vi "KeyDown.vi"(6 "PlatMods":T9, 7 "Type":T1, 8 "error in (no error)":errorcluster, 9 "VKey":T10, 10 "Char":i16, 11 "Data in":T2={"Class"={"Ants"=refnum, "Layer"=refnum, "Templates"=refnum, "Icon"=refnum, "Glyph"=refnum, "Settings"=refnum, "Tools"=refnum, "History"=refnum}, "Ref"={"Add Layer"=refnum, "Remove Layer"=refnum, "Line Text"=[], "Body Text Spec"=refnum, "DNL_Font"=refnum, "glyph path str"=refnum, "templates path str"=refnum, "Arrow Up"=refnum, "Arrow Down"=refnum, "IE VI Ref"=refnum, "Glyphs tree"=refnum, "Templates tree"=refnum, "Layer Icon Text"=refnum, "Layer Template"=refnum, "Body Text"=refnum, "Search Templates"=refnum, "TextMarker"=refnum, "Tab Control"=refnum, "Search Glyphs"=refnum, "Line Color"=refnum, "DNL_Glyphs []"=refnum, "Fill Color"=refnum, "Tools"=refnum, "Icon"=refnum, "Preview"=refnum, "Ants"=refnum, "Terminals"=refnum, "menu reference"=refnum, "LayerNames"=[], "GlyphLoadAnimation"=refnum, "TemplateLoadAnimation"=refnum, "refreshGlyphs"=refnum, "refreshTemplates"=refnum}, "Support"={"AntsRect"={"left"=0, "top"=0, "right"=0, "bottom"=0}, "Mouse Move Coords"={"Horizontal"=0, "Vertical"=0}, "Mouse Down Coords"={"Horizontal"=0, "Vertical"=0}, "Temp Coord"={"Horizontal"=0, "Vertical"=0}, "Action"=enum."Default", "Edge Color"=4914962, "Fill Color"=16860, "Mouse Down?"=FALSE, "Draft Mode?"=FALSE, "Temp Icon"=bytes[3102], "CTRL Pressed"=FALSE, "Move Selection?"=FALSE, "AntsRect Orig"={"left"=0, "top"=0, "right"=0, "bottom"=0}, "Text"="", "TM Set?"=FALSE, "Mouse inside icon?"=FALSE, "Tool (old value)"=0, "Pencil Move Color"=0, "Swap Colors?"=FALSE, "Shift pressed?"=FALSE}}) -> (0 "error out":errorcluster, 1 "Discard?":bool, 3 "Data out":T2={"Class"={"Ants"=refnum, "Layer"=refnum, "Templates"=refnum, "Icon"=refnum, "Glyph"=refnum, "Settings"=refnum, "Tools"=refnum, "History"=refnum}, "Ref"={"Add Layer"=refnum, "Remove Layer"=refnum, "Line Text"=[], "Body Text Spec"=refnum, "DNL_Font"=refnum, "glyph path str"=refnum, "templates path str"=refnum, "Arrow Up"=refnum, "Arrow Down"=refnum, "IE VI Ref"=refnum, "Glyphs tree"=refnum, "Templates tree"=refnum, "Layer Icon Text"=refnum, "Layer Template"=refnum, "Body Text"=refnum, "Search Templates"=refnum, "TextMarker"=refnum, "Tab Control"=refnum, "Search Glyphs"=refnum, "Line Color"=refnum, "DNL_Glyphs []"=refnum, "Fill Color"=refnum, "Tools"=refnum, "Icon"=refnum, "Preview"=refnum, "Ants"=refnum, "Terminals"=refnum, "menu reference"=refnum, "LayerNames"=[], "GlyphLoadAnimation"=refnum, "TemplateLoadAnimation"=refnum, "refreshGlyphs"=refnum, "refreshTemplates"=refnum}, "Support"={"AntsRect"={"left"=0, "top"=0, "right"=0, "bottom"=0}, "Mouse Move Coords"={"Horizontal"=0, "Vertical"=0}, "Mouse Down Coords"={"Horizontal"=0, "Vertical"=0}, "Temp Coord"={"Horizontal"=0, "Vertical"=0}, "Action"=enum."Default", "Edge Color"=4914962, "Fill Color"=16860, "Mouse Down?"=FALSE, "Draft Mode?"=FALSE, "Temp Icon"=bytes[3102], "CTRL Pressed"=FALSE, "Move Selection?"=FALSE, "AntsRect Orig"={"left"=0, "top"=0, "right"=0, "bottom"=0}, "Text"="", "TM Set?"=FALSE, "Mouse inside icon?"=FALSE, "Tool (old value)"=0, "Pencil Move Color"=0, "Swap Colors?"=FALSE, "Shift pressed?"=FALSE}})   [LabVIEW 2020]
uses:
  Class/Ants/Ants.lvclass
  Class/FakedArray/FakedArray.lvclass
  vi.lib/LabVIEW Icon API/lv_icon/Classes/Icon/Icon.lvclass
  Class/Icon Library/Glyph.lvclass
  Class/Settings/Settings.lvclass
  Class/Tools/Tools Paint.lvclass
  History/History/History.lvclass
  lv_icon.lvlib
  <vilib>/Utility/miscctls.llb/LVPoint32TypeDef.ctl
  <vilib>/event_ctls.llb/lveventtype.ctl
  Controls/SupportClass_Action.ctl
  History/History.lvlib
  <vilib>/event_ctls.llb/eventvkey.ctl
  Controls/Support Cluster.ctl
  Controls/References Cluster.ctl
  Controls/IE Classes.ctl
  Controls/Global Data.ctl
  vi.lib/LabVIEW Icon API/lv_icon/Controls/IEColor.ctl
panel:
  in  "Layer name":string="Clipboard"
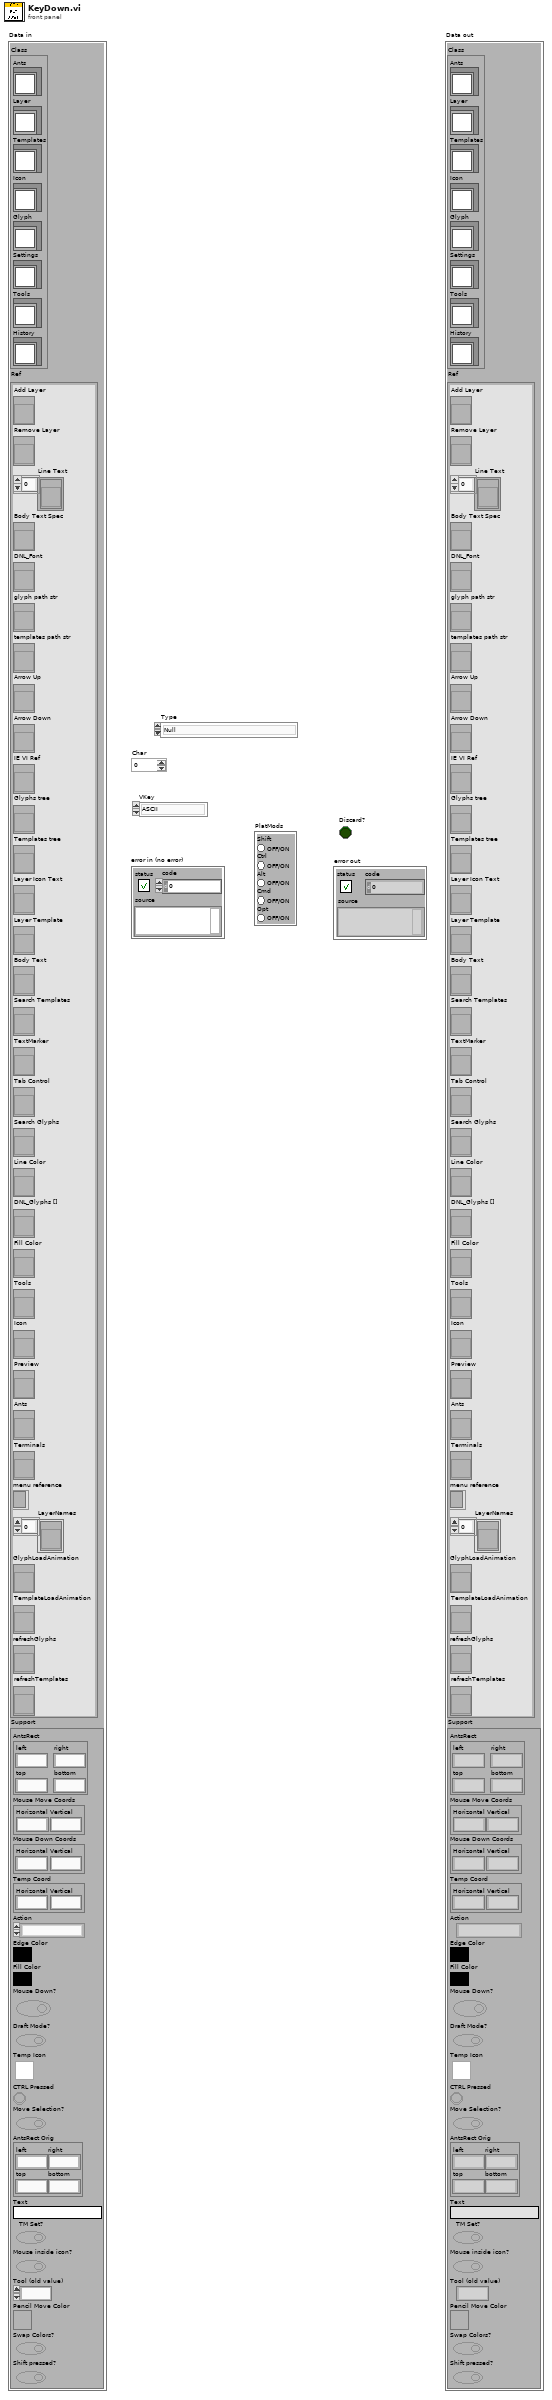
[diagram p1: front panel]
types:
  T1 = typedef "lveventtype.ctl" = enum32{"Null", "Timeout", "Annotation Menu Selection", "Annotation Menu Selection?", "App Instance Close", "App Instance Close?", "Autoscale Range Change", "Bookmark Info Change", "Cell Edit", "Cell Edit?", "Cursor Grab", "Cursor Grab?", "Cursor Menu Selection", "Cursor Menu Selection?", "Cursor Move", "Cursor Release", "Data Change", "Direction Change", "Display State Change", "Drag Ended", "Drag Enter", "Drag Leave", "Drag Over", "Drag Source Update", "Drag Starting", "Drag Starting?", "Drop", "Exec State Change", "Key Down", "Key Down?", "Key Repeat", "Key Repeat?", "Key Up", "Listbox Double Click", "Menu Activation?", "Menu Selection (App)", "Menu Selection? (App)", "Menu Selection (User)", "Mouse Down", "Mouse Down?", "Mouse Enter", "Mouse Leave", "Mouse Move", "Mouse Up", "Mouse Wheel", "NI Security User Change (App)", "Pane Size", "Panel Close", "Panel Close?", "Panel Resize", "Plot Attribute Change", "Scale Range Change", "Shortcut Menu Activation?", "Shortcut Menu Selection (App)", "Shortcut Menu Selection? (App)", "Shortcut Menu Selection (User)", "Tree Double Click", "Tree Drag", "Tree Drag?", "Tree Drop", "Tree Drop?", "Tree Item Close", "Tree Item Close?", "Tree Item Open", "Tree Item Open?", "URL Change?", "User Event", "Value Change"}
  T2 = typedef "lv_icon.lvlib/Global Data.ctl" = cluster{"Class":T3, "Ref":T4, "Support":T5}
  T3 = typedef "lv_icon.lvlib/IE Classes.ctl" = cluster{"Ants":refnum<class "Ants.lvclass">, "Layer":refnum<class "FakedArray.lvclass">, "Templates":refnum<class "FakedArray.lvclass">, "Icon":refnum<class "Icon.lvclass">, "Glyph":refnum<class "Glyph.lvclass">, "Settings":refnum<class "Settings.lvclass">, "Tools":refnum<class "Tools Paint.lvclass">, "History":refnum<class "History.lvclass">}
  T4 = typedef "lv_icon.lvlib/References Cluster.ctl" = cluster{"Add Layer":refnum<vi>, "Remove Layer":refnum<vi>, "Line Text":refnum<vi>[], "Body Text Spec":refnum<vi>, "DNL_Font":refnum<vi>, "glyph path str":refnum<vi>, "templates path str":refnum<vi>, "Arrow Up":refnum<vi>, "Arrow Down":refnum<vi>, "IE VI Ref":refnum<vi>, "Glyphs tree":refnum<vi>, "Templates tree":refnum<vi>, "Layer Icon Text":refnum<vi>, "Layer Template":refnum<vi>, "Body Text":refnum<vi>, "Search Templates":refnum<vi>, "TextMarker":refnum<vi>, "Tab Control":refnum<vi>, "Search Glyphs":refnum<vi>, "Line Color":refnum<vi>, "DNL_Glyphs []":refnum<vi>, "Fill Color":refnum<vi>, "Tools":refnum<vi>, "Icon":refnum<vi>, "Preview":refnum<vi>, "Ants":refnum<vi>, "Terminals":refnum<vi>, "menu reference":refnum<k9>, "LayerNames":refnum<vi>[], "GlyphLoadAnimation":refnum<vi>, "TemplateLoadAnimation":refnum<vi>, "refreshGlyphs":refnum<vi>, "refreshTemplates":refnum<vi>}
  T5 = typedef "lv_icon.lvlib/Support Cluster.ctl" = cluster{"AntsRect":cluster{"left":i16, "top":i16, "right":i16, "bottom":i16}, "Mouse Move Coords":T6, "Mouse Down Coords":T6, "Temp Coord":T6, "Action":T7, "Edge Color":T8, "Fill Color":T8, "Mouse Down?":bool, "Draft Mode?":bool, "Temp Icon":picture, "CTRL Pressed":bool, "Move Selection?":bool, "AntsRect Orig":cluster{"left":i16, "top":i16, "right":i16, "bottom":i16}, "Text":string, "TM Set?":bool, "Mouse inside icon?":bool, "Tool (old value)":u32, "Pencil Move Color":u32, "Swap Colors?":bool, "Shift pressed?":bool}
  T6 = typedef "LVPoint32TypeDef.ctl" = cluster{"Horizontal":i32, "Vertical":i32}
  T7 = typedef "SupportClass_Action.ctl" = enum16{"Default", "Move Selection", "Glyph Library", "Tool"}
  T8 = typedef "IEColor.ctl" = u32
  T9 = cluster{"Shift":bool, "Ctrl":bool, "Alt":bool, "Cmd":bool, "Opt":bool}
  T10 = typedef "eventvkey.ctl" = enum16{"ASCII", "Enter", "Return", "Shift", "Ctrl", "Alt", "Cmd", "Opt", "Caps", "NumLock", "Clear", "Break", "Up", "Down", "Left", "Right", "Insert", "Delete", "Home", "End", "PageUp", "PageDown", "Escape", "Help", "Pause", "ScrollLock", "F1", "F2", "F3", "F4", "F5", "F6", "F7", "F8", "F9", "F10", "F11", "F12", "F13", "F14", "F15", "F16", "F17", "F18", "F19", "F20", "F21", "F22", "F23", "F24", "Play", "VolumeUp", "VolumeDown", "Mute", "Two Byte Char"}
  T11 = cluster{"left":i16, "top":i16, "right":i16, "bottom":i16}
  T12 = enum32{"Pencil", "Line", "Dropper", "Fill", "Rectangle", "Filled Rectangle", "Ellipse", "Filled Ellipse", "Eraser", "Text", "Select", "Move"}
  T13 = typedef "Graphic.ctl" = cluster{"Rectangle":cluster{"left":i16, "top":i16, "right":i16, "bottom":i16}, "Path":path, "Image":picture, "Filter":string, "FileName":string}
  T14 = cluster{"left":i16, "top":i16, "bottom":i16, "right":i16}
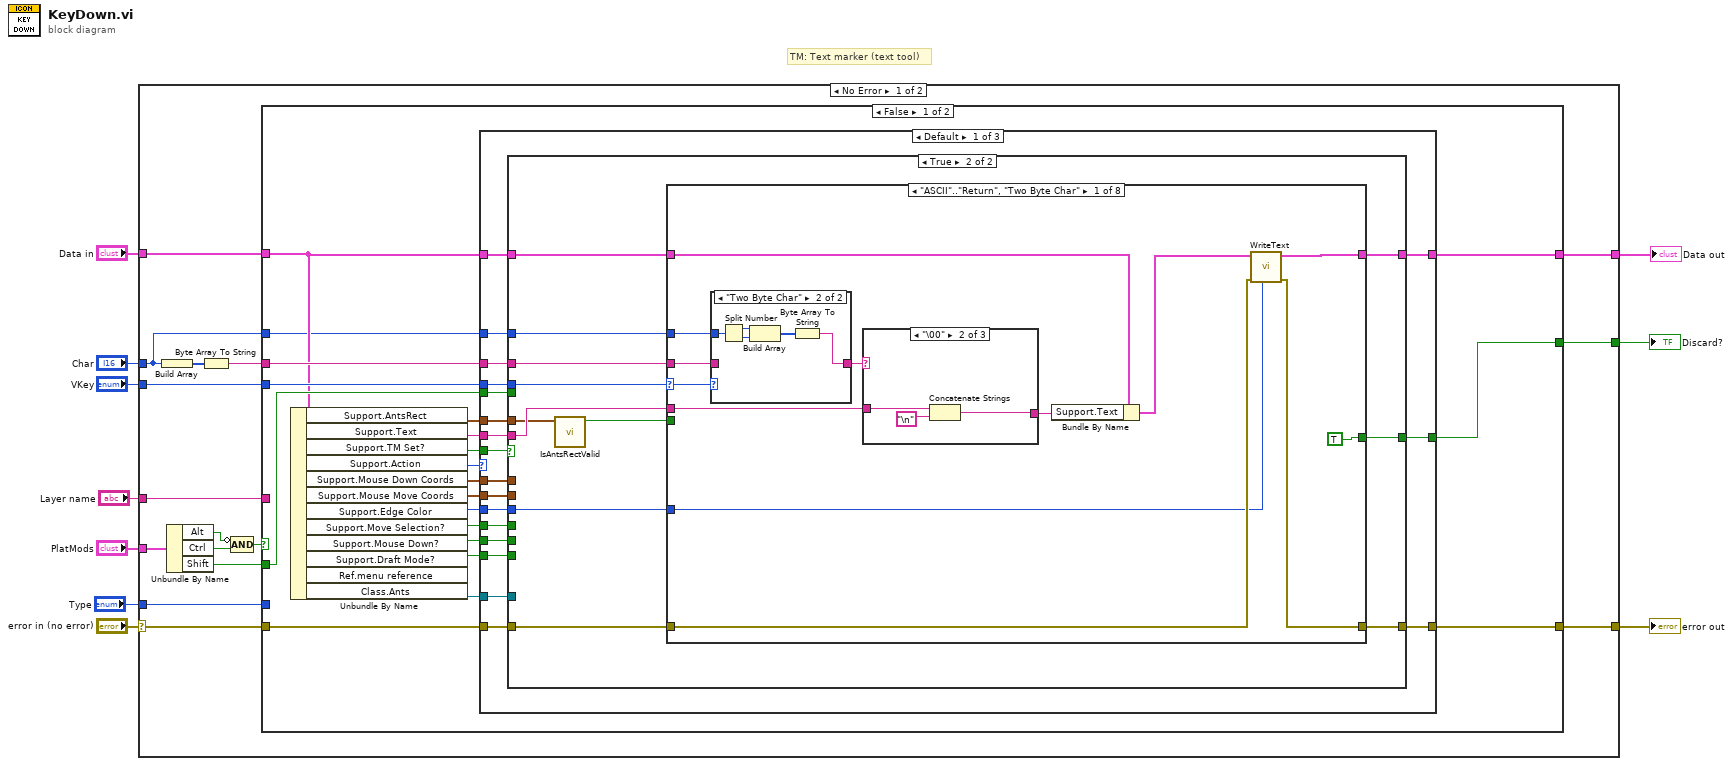
[diagram p0: block diagram]
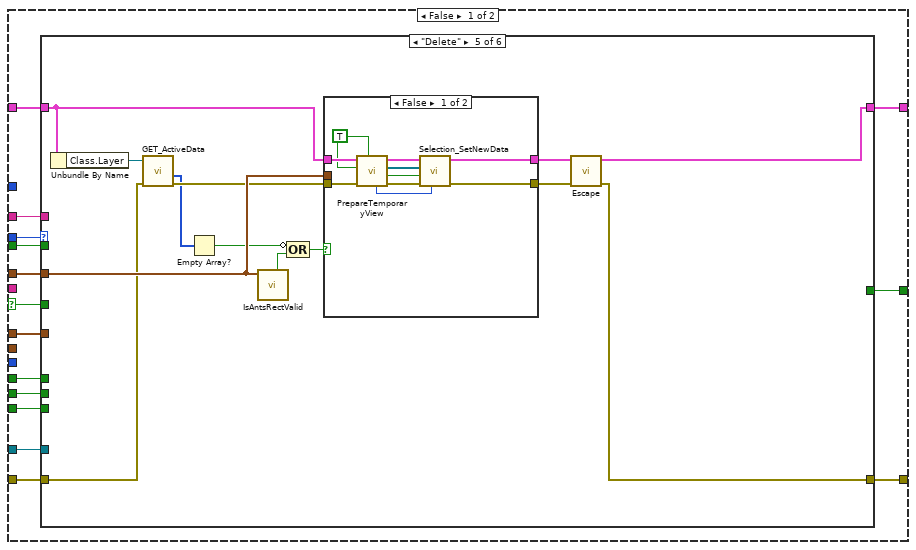
[diagram p2: hidden frame]
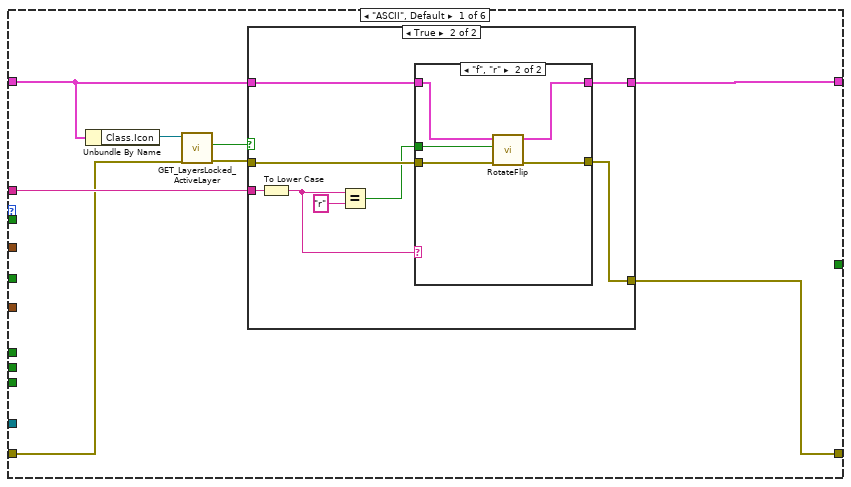
[diagram p3: hidden frame]
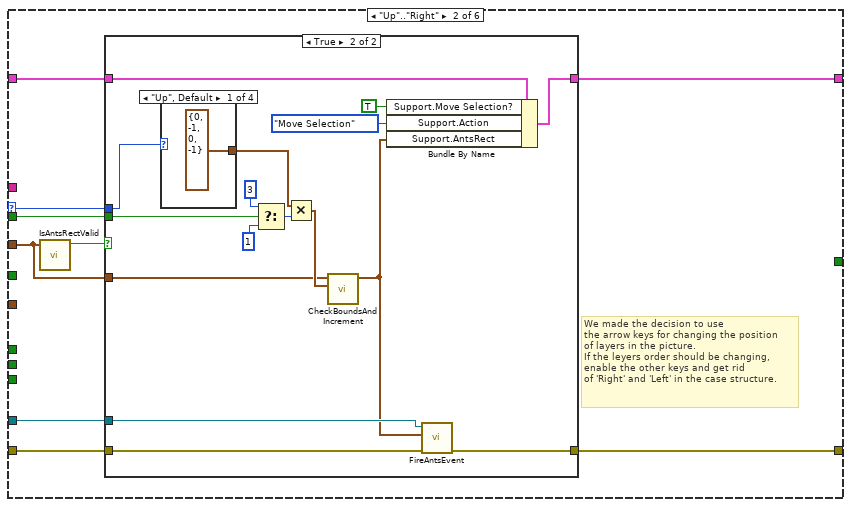
[diagram p6: hidden frame]
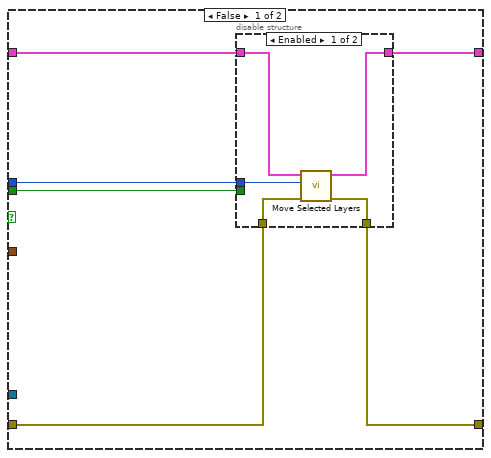
[diagram p7: hidden frame]
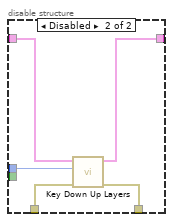
[diagram p8: hidden frame]
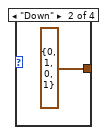
[diagram p9: hidden frame]
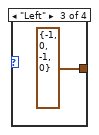
[diagram p10: hidden frame]
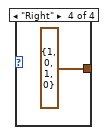
[diagram p11: hidden frame]
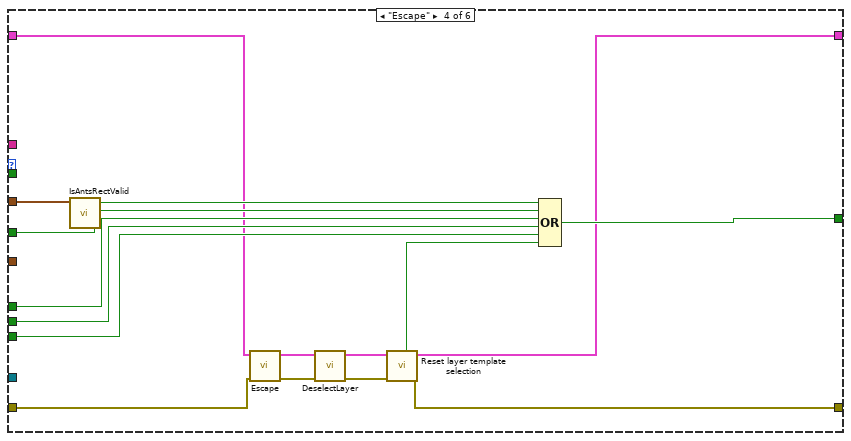
[diagram p13: hidden frame]
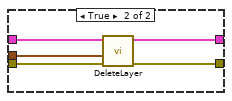
[diagram p14: hidden frame]
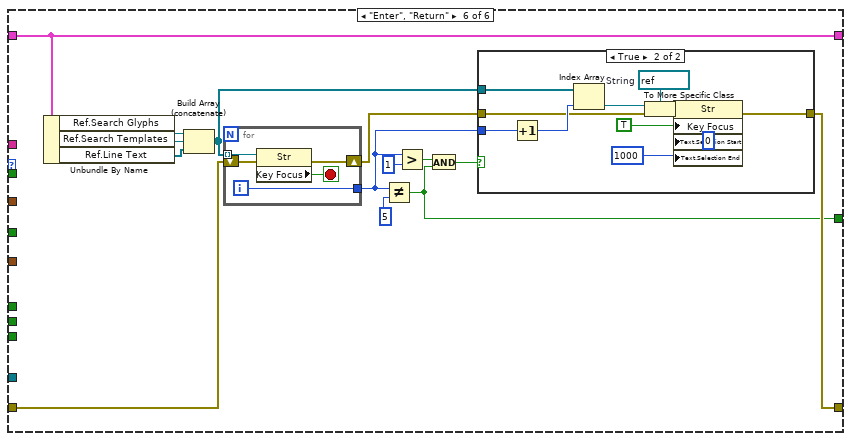
[diagram p15: hidden frame]
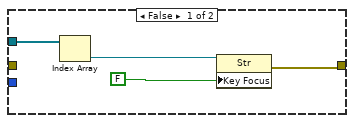
[diagram p16: hidden frame]
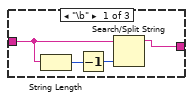
[diagram p18: hidden frame]
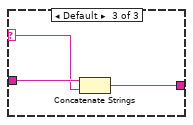
[diagram p19: hidden frame]
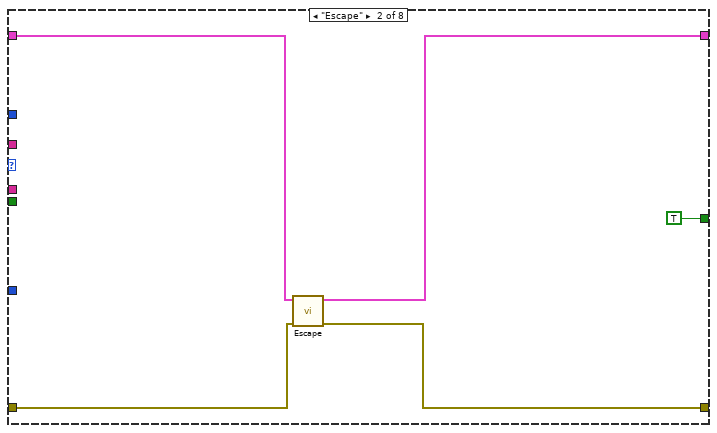
[diagram p20: hidden frame]
diagram:
  # "TM: Text marker (text tool)"
  n1 = case shown="No Error" "error in (no error)" {
    selector: "error in (no error)" -> [w21 w703]
    tunnel: [w23 w703] -> w9
    tunnel: "VKey" -> [w26 _]
    tunnel: "Char" -> [w18 _]
    tunnel: "PlatMods" -> [w15 _]
    tunnel: [w22 _] -> w5
    tunnel: "Data in" -> [w16 w702]
    tunnel: [w20 w702] -> w3
    tunnel: "Type" -> [w19 _]
    tunnel: "Layer name" -> [w17 _]
    frame No Error {
      n2 = Build Array(w18) -> (w25:i16[])
      n3 = Unbundle By Name(w15) -> ("Alt"=w11:bool, "Ctrl"=w14:bool, "Shift"=w13:bool)
      n4 = Byte Array To String(unsigned byte array=w25) -> (string=w24:string)
      n5 = Compound Arithmetic op=AND(invert w11, w14) -> (w12:bool)
      n6 = case shown="False" w12 {
        selector: w12 -> [_ w493]
        tunnel: w26 -> [w46 _]
        tunnel: w24 -> [w45 w491]
        tunnel: [w30 w503] -> w23
        tunnel: [w34 w490] -> w22
        tunnel: w21 -> [w32 w506]
        tunnel: w13 -> [w33 w494]
        tunnel: w16 -> [w31 w505]
        tunnel: [w28 w504] -> w20
        tunnel: w19 -> [_ w498]
        tunnel: w18 -> [w27 _]
        tunnel: w17 -> [_ w488]
        frame False {
          n7 = Unbundle By Name(w31) -> ("Support.AntsRect"=w39:T11, "Support.Text"=w42:string, "Support.TM Set?"=w43:bool, "Support.Action"=w44:T7, "Support.Mouse Down Coords"=w41:T6, "Support.Mouse Move Coords"=w38:T6, "Support.Edge Color"=w40:T8, "Support.Move Selection?"=w37:bool, "Support.Mouse Down?"=w36:bool, "Support.Draft Mode?"=w35:bool, "Class.Ants"=w29:refnum<class "Ants.lvclass">)  [unwired: 1 out]
          n8 = case shown="Default" w44 {
            tunnel: w46 -> [w65 w339 w406]
            tunnel: w45 -> [w60 w338 _]
            tunnel: w32 -> [w63 w337 w408]
            tunnel: [w64 w336 w407] -> w30
            tunnel: w43 -> [w62 w334 w404]
            tunnel: w42 -> [w61 _ _]
            tunnel: w41 -> [w59 _ _]
            tunnel: w40 -> [w58 _ _]
            tunnel: w39 -> [w57 w335 w405]
            tunnel: w38 -> [w56 w327 _]
            tunnel: w37 -> [w55 w333 w403]
            tunnel: w36 -> [w54 w332 w402]
            tunnel: w35 -> [w53 w331 w401]
            tunnel: [w52 w330 w400] -> w34
            tunnel: w33 -> [w51 _ w396]
            tunnel: w31 -> [w50 w329 w399]
            tunnel: [w49 w328 w398] -> w28
            tunnel: w29 -> [w47 _ w397]
            tunnel: w27 -> [w48 _ _]
            frame Default {
              n9 = case shown="True" w62 {
                selector: w62 -> [w71 _]
                tunnel: w65 -> [w79 w242]
                tunnel: [w78 w241] -> w64
                tunnel: w63 -> [w80 w240]
                tunnel: w61 -> [_ w239]
                tunnel: w60 -> [w77 w238]
                tunnel: w59 -> [w75 _]
                tunnel: w58 -> [_ w235]
                tunnel: w57 -> [w76 w237]
                tunnel: w56 -> [_ _]
                tunnel: w55 -> [w74 _]
                tunnel: w54 -> [w73 _]
                tunnel: w53 -> [w72 _]
                tunnel: [w70 w234] -> w52
                tunnel: w51 -> [w69 _]
                tunnel: w50 -> [w68 w233]
                tunnel: [w67 w232] -> w49
                tunnel: w48 -> [_ w231]
                tunnel: w47 -> [w66 _]
                frame False {
                  n10 = case shown="\"Delete\"" w79 {
                    selector: w79 -> [_ w112 _ _ _ _]
                    tunnel: w80 -> [w84 w114 w152 w168 w175 w209]
                    tunnel: [w87 w113 w152 w165 w181 w206] -> w78
                    tunnel: w77 -> [w88 _ _ _ _ _]
                    tunnel: w76 -> [_ w107 _ w163 w178 _]
                    tunnel: w75 -> [_ _ _ _ _ _]
                    tunnel: w74 -> [_ _ _ w161 _ _]
                    tunnel: w73 -> [_ _ _ w160 _ _]
                    tunnel: w72 -> [_ _ _ w159 _ _]
                    tunnel: w71 -> [_ _ _ w162 _ _]
                    tunnel: [_ _ _ w158 _ w198] -> w70
                    tunnel: w69 -> [_ w111 _ _ _ _]
                    tunnel: w68 -> [w86 w110 w151 w156 w176 w210]
                    tunnel: [w85 w109 w151 w153 w180 w210] -> w67
                    tunnel: w66 -> [_ w106 _ _ _ _]
                    frame "ASCII", Default {
                      n11 = Unbundle By Name(w86) -> ("Class.Icon"=w82:refnum<class "Icon.lvclass">)
                      n12 = call-dynamic "GET_LayersLocked_ActiveLayer.vi"("error in (no error)"=w84, "Icon.lvclass in"=w82) -> ("error out"=w83:errorcluster, "Layers Locked?"=w81:bool)  [unwired: 8 out]
                      n13 = case shown="True" w81 {
                        tunnel: w88 -> [_ w95]
                        tunnel: w83 -> [w90 w98]
                        tunnel: [w90 w97] -> w87
                        tunnel: w86 -> [w89 w92]
                        tunnel: [w89 w91] -> w85
                        frame False {
                        }
                        frame True {
                          n14 = To Lower Case(string=w95) -> (all lower case string=w93:string)
                          n15 = Equal?(x=w93, y="r") -> (x = y?=w94:bool)
                          n16 = case shown="\"f\", \"r\"" w93 {
                            tunnel: w98 -> [w100 w105]
                            tunnel: [w100 w103] -> w97
                            tunnel: w94 -> [_ w104]
                            tunnel: w92 -> [w99 w102]
                            tunnel: [w99 w101] -> w91
                            frame Default {
                            }
                            frame "f", "r" {
                              n17 = call "RotateFlip.vi"("error in"=w105, "Rotate"=w104, "Data in"=w102) -> ("error out"=w103:errorcluster, "Data out"=w101:T2)  [unwired: 3 in, 4 out]
                            }
                          }
                        }
                      }
                    }
                    frame "Up".."Right" {
                      # "We made the decision to use\nthe arrow keys for changing the position\nof layers in the picture.\nIf the leyers order should be changing,\nenable the other keys and get rid\nof 'Right' and 'Left' in the case structure."
                      n18 = call "IsAntsRectValid.vi"("AntsRect"=w107) -> ("Valid?"=w108:bool)  [unwired: 10 out]
                      n19 = case shown="True" w108 {
                        tunnel: w114 -> [w120 w131]
                        tunnel: [w119 w135] -> w113
                        tunnel: w112 -> [w118 w137]
                        tunnel: w111 -> [w117 w136]
                        tunnel: w110 -> [w116 w145]
                        tunnel: [w115 w143] -> w109
                        tunnel: w107 -> [_ w133]
                        tunnel: w106 -> [_ w134]
                        frame False {
                          n20 = disable-structure shown="Enabled" {
                            disable-tunnel: w120 -> [w123 w128]
                            disable-tunnel: [w122 w127] -> w119
                            disable-tunnel: w118 -> [w121 w126]
                            disable-tunnel: w117 -> [_ _]
                            disable-tunnel: w116 -> [w125 w130]
                            disable-tunnel: [w124 w129] -> w115
                            frame Enabled {
                              n21 = call "Move Selected Layers.vi"("error in"=w123, "VKey"=w121, "Data in"=w125) -> ("error out"=w122:errorcluster, "Data out"=w124:T2)  [unwired: 1 in, 6 out]
                            }
                            frame Disabled {
                              n22 = call "Key Down Up Layers.vi"("error in"=w128, "VKey"=w126, "Data in"=w130) -> ("error out"=w127:errorcluster, "Data out"=w129:T2)  [unwired: 1 in, 6 out]
                            }
                          }
                        }
                        frame True {
                          n23 = case shown="\"Up\", Default" w137 {
                            tunnel: [T11 {"left"=0, "top"=-1, "right"=0, "bottom"=-1} ("y") T11 {"left"=0, "top"=1, "right"=0, "bottom"=1} ("y") T11 {"left"=-1, "top"=0, "right"=-1, "bottom"=0} ("y") T11 {"left"=1, "top"=0, "right"=1, "bottom"=0} ("y")] -> w141
                            frame "Up", Default {
                            }
                            frame "Down" {
                            }
                            frame "Left" {
                            }
                            frame "Right" {
                            }
                          }
                          n24 = Select(t=i16 3 ("left"), s=w136, f=i16 1 ("left")) -> (s? t:f=w138:i16)
                          n25 = Multiply(x=w141, y=w138) -> (x*y=w146:T11)
                          n26 = call "CheckBoundsAndIncrement.vi"("Increment"=w146, "Rectangle In"=w133) -> ("Rectangle Out"=w132:T11)  [unwired: 9 in]
                          n27 = Bundle By Name(cluster=w145, "Support.Move Selection?"=TRUE, "Support.Action"=SupportClass_Action."Move Selection", "Support.AntsRect"=w132) -> (w143:T2)
                          n28 = call "FireAntsEvent.vi"("error in (no error)"=w131, "Rectangle (default: deselect)"=w132, "Ants in"=w134) -> ("error out"=w135:errorcluster)  [unwired: 1 in, 7 out]
                        }
                      }
                    }
                    frame "Shift" {
                    }
                    frame "Escape" {
                      n29 = call "IsAntsRectValid.vi"("AntsRect"=w163) -> ("Valid?"=w164:bool)  [unwired: 10 out]
                      n30 = call "Escape.vi"("error in"=w168, "Data in"=w156) -> ("error out"=w167:errorcluster, "Data out"=w155:T2)  [unwired: 8 out]
                      n31 = call "DeselectLayer.vi"("error in (no error)"=w167, "Data in"=w155) -> ("error out"=w166:errorcluster, "Data out"=w154:T2)  [unwired: 8 out]
                      n32 = call "Reset layer template selection.vi"("error in (no error)"=w166, "Data in"=w154) -> ("error out"=w165:errorcluster, "Data out"=w153:T2, "Layers selected?"=w157:bool)  [unwired: 1 in, 6 out]
                      n33 = Compound Arithmetic op=OR(w164, w162, w161, w160, w159, w157) -> (w158:bool)
                    }
                    frame "Delete" {
                      n34 = Unbundle By Name(w176) -> ("Class.Layer"=w177:refnum<class "FakedArray.lvclass">)
                      n35 = call-dynamic "GET_ActiveData.vi"("error in (no error)"=w175, "FakedArray in"=w177) -> ("error out"=w174:errorcluster, "Active Data []"=w173:i32[])  [unwired: 4 in, 4 out]
                      n36 = Empty Array?(array=w173) -> (empty?=w171:bool)
                      n37 = call "IsAntsRectValid.vi"("AntsRect"=w178) -> ("Max. Rect size?"=w172:bool)  [unwired: 10 out]
                      n38 = Compound Arithmetic op=OR(invert w171, w172) -> (w170:bool)
                      n39 = case shown="False" w170 {
                        tunnel: w176 -> [w191 w196]
                        tunnel: [w190 w194] -> w179
                        tunnel: [w189 w195] -> w169
                        tunnel: w174 -> [w182 w193]
                        tunnel: w178 -> [_ w192]
                        frame False {
                          w188 = TRUE ("Delete Selected Area?")
                          n40 = call "PrepareTemporaryView.vi"("Delete Selected Area?"=w188, "error in (no error)"=w182, "Valid Selection?"=w188, "Data in"=w191) -> ("error out"=w185:errorcluster, "Highlighted?"=w186:bool, "All Layers out"=w187:refnum<class "Layer.lvclass">[], "Data out"=w183:T2, "#Active Layer"=w184:i32)  [unwired: 1 in, 2 out]
                          n41 = call "Selection_SetNewData.vi"("#Active Layer"=w184, "error in"=w185, "Highlighted?"=w186, "All Layers In"=w187, "Data in"=w183) -> ("error out"=w190:errorcluster, "Data out"=w189:T2)  [unwired: 1 in, 3 out]
                        }
                        frame True {
                          n42 = call "DeleteLayer.vi"("error in"=w193, "AntsRect"=w192, "Data in"=w196) -> ("error out"=w194:errorcluster, "Data out"=w195:T2)  [unwired: 5 out]
                        }
                      }
                      n43 = call "Escape.vi"("error in"=w179, "Data in"=w169) -> ("error out"=w181:errorcluster, "Data out"=w180:T2)  [unwired: 8 out]
                    }
                    frame "Enter", "Return" {
                      n44 = Unbundle By Name(w210) -> ("Ref.Search Glyphs"=w202:refnum<vi>, "Ref.Search Templates"=w203:refnum<vi>, "Ref.Line Text"=w205:refnum<vi>[])
                      n45 = Build Array (concatenate)(w202, w203, w205) -> (w204:refnum<vi>[])
                      n46 = for {
                        tunnel: w204 -> [w230] mode=indexing
                        shift-right: [w229] -> w207
                        shift-left: w209 -> [w228]
                        tunnel: [w227] -> w201
                        i -> [w227]
                        stop <- w226 stop-if-true
                        n47 = property class="Str"(reference=w230, error in=w228) -> (error out=w229:errorcluster, "Key Focus"=w226:bool)  [unwired: 1 out]
                      }
                      n48 = Not Equal?(x=w201, y=5) -> (x != y?=w198:bool)
                      n49 = Greater?(x=w201, y=1) -> (0:w199:bool)
                      n50 = And(x=w199, y=w198) -> (x .and. y?=w197:bool)
                      n51 = case shown="True" w197 {
                        tunnel: w201 -> [_ w224]
                        tunnel: w204 -> [w214 w225]
                        tunnel: w207 -> [_ w221]
                        tunnel: [w211 w219] -> w206
                        frame False {
                          n52 = Index Array(array=w214) -> (element=w213:refnum<vi>)  [unwired: 1 in]
                          n53 = property class="Str"(reference=w213, "Key Focus"=FALSE) -> (error out=w211:errorcluster)  [unwired: 1 in, 1 out]
                        }
                        frame True {
                          w215 = refnum<vi> refnum  # String
                          n54 = Increment(x=w224) -> (x+1=w223:i32)
                          n55 = Index Array(array=w225, index=w223) -> (element=w222:refnum<vi>)
                          n56 = To More Specific Class(target class=w215, reference=w222) -> (specific class reference=w216:refnum<vi>)  [unwired: 1 in, 1 out]
                          n57 = property class="Str"(reference=w216, error in=w221, "Key Focus"=TRUE, "Text.Selection Start"=u32 0 ("Text.Selection:Start"), "Text.Selection End"=u32 1000 ("Text.Selection:End")) -> (error out=w219:errorcluster)  [unwired: 1 out]
                        }
                      }
                    }
                  }
                }
                frame True {
                  n58 = call "IsAntsRectValid.vi"("AntsRect"=w237) -> ("Valid?"=w236:bool)  [unwired: 10 out]
                  n59 = case shown="\"ASCII\"..\"Return\", \"Two Byte Char\"" w242 {
                    selector: w242 -> [w246 _ _ _ _ _ _ _]
                    tunnel: [w253 w275 w278 w282 w306 w312 w318 w324] -> w241
                    tunnel: w240 -> [w254 w276 w278 w283 w307 w313 w319 w325]
                    tunnel: w239 -> [w255 _ _ w284 _ _ _ _]
                    tunnel: w238 -> [w244 _ _ _ _ _ _ _]
                    tunnel: w235 -> [w252 _ _ _ w308 w314 w320 w326]
                    tunnel: w236 -> [_ _ _ w281 _ _ _ _]
                    tunnel: [TRUE TRUE _ _ _ _ _ _] -> w234
                    tunnel: w233 -> [w247 w273 w277 w280 w305 w310 w317 w323]
                    tunnel: [w250 w272 w277 w279 w303 w309 w316 w321] -> w232
                    tunnel: w231 -> [w243 _ _ _ _ _ _ _]
                    frame "ASCII".."Return", "Two Byte Char" {
                      n60 = case shown="\"Two Byte Char\"" w246 {
                        tunnel: [w256 w257] -> w245
                        tunnel: w244 -> [w256 _]
                        tunnel: w243 -> [_ w261]
                        frame "ASCII", Default {
                        }
                        frame "Two Byte Char" {
                          n61 = Split Number(x=w261) -> (hi(x)=w259:u8, lo(x)=w260:u8)
                          n62 = Build Array(w259, w260) -> (w258:u8[])
                          n63 = Byte Array To String(unsigned byte array=w258) -> (string=w257:string)
                        }
                      }
                      n64 = case shown="\"\\00\"" w245 {
                        selector: w245 -> [_ _ w269]
                        tunnel: w255 -> [w263 w268 w271]
                        tunnel: [w262 w267 w270] -> w249
                        frame "\b" {
                          n65 = String Length(string=w263) -> (length=w265:i32)
                          n66 = Decrement(x=w265) -> (x-1=w264:i32)
                          n67 = Search/Split String(string=w263, offset (0)=w264) -> (substring before match=w262:string)  [unwired: 3 out]
                        }
                        frame "\u0000\u0000" {
                          n68 = Concatenate Strings(w268, "\n") -> (w267:string)
                        }
                        frame Default {
                          n69 = Concatenate Strings(w271, w269) -> (w270:string)
                        }
                      }
                      n70 = Bundle By Name(cluster=w247, "Support.Text"=w249) -> (w248:T2)
                      n71 = call "WriteText.vi"("Text Color"=w252, "error in (no error)"=w254, "Data in"=w248) -> ("error out"=w253:errorcluster, "Data out"=w250:T2)  [unwired: 2 in, 5 out]
                    }
                    frame "Escape" {
                      n72 = call "Escape.vi"("error in"=w276, "Data in"=w273) -> ("error out"=w275:errorcluster, "Data out"=w272:T2)  [unwired: 8 out]
                    }
                    frame Default {
                    }
                    frame "Delete" {
                      n73 = case shown="True" w281 {
                        tunnel: w284 -> [_ _]
                        tunnel: w283 -> [w286 w295]
                        tunnel: [w286 w297] -> w282
                        tunnel: w280 -> [w285 w290]
                        tunnel: [w285 w292] -> w279
                        frame False {
                        }
                        frame True {
                          w302 = TRUE ("Delete Selected Area?")
                          n74 = call "PrepareTemporaryView.vi"("Delete Selected Area?"=w302, "error in (no error)"=w295, "Valid Selection?"=w302, "Data in"=w290) -> ("error out"=w298:errorcluster, "Highlighted?"=w300:bool, "All Layers out"=w301:refnum<class "Layer.lvclass">[], "Data out"=w294:T2, "#Active Layer"=w299:i32)  [unwired: 1 in, 2 out]
                          n75 = call "Selection_SetNewData.vi"("#Active Layer"=w299, "error in"=w298, "Highlighted?"=w300, "All Layers In"=w301, "Data in"=w294) -> ("error out"=w296:errorcluster, "Data out"=w293:T2)  [unwired: 1 in, 3 out]
                          n76 = call "ViewLayer.vi"("error in (no error)"=w296, "Data in"=w293) -> ("error out"=w291:errorcluster, "Data out"=w288:T2)  [unwired: 3 in, 5 out]
                          n77 = call "Set Undo Flag.vi"("error in"=w291, "Data in"=w288) -> ("error out"=w289:errorcluster, "Data out"=w287:T2)  [unwired: 8 in]
                          n78 = call "Escape.vi"("error in"=w289, "Data in"=w287) -> ("error out"=w297:errorcluster, "Data out"=w292:T2)  [unwired: 8 out]
                        }
                      }
                    }
                    frame "Up" {
                      n79 = call "WriteText.vi"("Text Color"=w308, "error in (no error)"=w307, "Offset"=T6 {"Horizontal"=0, "Vertical"=-1} ("y"), "Data in"=w305) -> ("error out"=w306:errorcluster, "Data out"=w303:T2)  [unwired: 1 in, 5 out]
                    }
                    frame "Down" {
                      n80 = call "WriteText.vi"("Text Color"=w314, "error in (no error)"=w313, "Offset"=T6 {"Horizontal"=0, "Vertical"=1} ("y"), "Data in"=w310) -> ("error out"=w312:errorcluster, "Data out"=w309:T2)  [unwired: 1 in, 5 out]
                    }
                    frame "Left" {
                      n81 = call "WriteText.vi"("Text Color"=w320, "error in (no error)"=w319, "Offset"=T6 {"Horizontal"=-1, "Vertical"=0} ("y"), "Data in"=w317) -> ("error out"=w318:errorcluster, "Data out"=w316:T2)  [unwired: 6 out]
                    }
                    frame "Right" {
                      n82 = call "WriteText.vi"("Text Color"=w326, "error in (no error)"=w325, "Offset"=T6 {"Horizontal"=1, "Vertical"=0} ("y"), "Data in"=w323) -> ("error out"=w324:errorcluster, "Data out"=w321:T2)  [unwired: 6 out]
                    }
                  }
                }
              }
            }
            frame "Glyph Library" {
              n83 = case shown="\"Escape\"" w339 {
                tunnel: w337 -> [w344 w391 w394]
                tunnel: [w343 w390 w394] -> w336
                tunnel: w338 -> [w345 _ _]
                tunnel: w335 -> [_ w388 _]
                tunnel: w334 -> [_ w387 _]
                tunnel: w333 -> [_ w386 _]
                tunnel: w332 -> [_ w385 _]
                tunnel: w331 -> [_ w384 _]
                tunnel: [_ w383 _] -> w330
                tunnel: w329 -> [w342 w382 w393]
                tunnel: [w341 w380 w392] -> w328
                tunnel: w327 -> [w340 _ _]
                frame "ASCII", Default {
                  n84 = case shown="Default" w345 {
                    selector: w345 -> [_ w364]
                    tunnel: w344 -> [w347 w350]
                    tunnel: [w347 w349] -> w343
                    tunnel: w342 -> [w346 w354]
                    tunnel: [w346 w351] -> w341
                    tunnel: w340 -> [_ w348]
                    frame Default {
                    }
                    frame "F", "R", "f", "r" {
                      n85 = Unbundle By Name(w354) -> ("Class.Glyph"=w355:refnum<class "Glyph.lvclass">)
                      n86 = call-dynamic "GET_ActiveGlyph.vi"("error in (no error)"=w350, "Glyph.lvclass in"=w355) -> ("error out"=w367:errorcluster, "Path & Icon"=w369:T13, "Glyph.lvclass out"=w368:refnum<class "Glyph.lvclass">)  [unwired: 7 out]
                      n87 = Unbundle By Name(w369) -> ("Image"=w371:picture, "Rectangle"=w370:T11)
                      n88 = Equal?(x=w364, y="r") -> (x = y?=w361:bool)
                      n89 = Equal?(x=w364, y="R") -> (x = y?=w362:bool)
                      n90 = Or(x=w361, y=w362) -> (x .or. y?=w356:bool)
                      n91 = call "Rotate Flip Image.vi"("Rotate?"=w356, "rect"=w370, "Temp Icon In"=w371) -> ("rect out"=w359:T14, "Temp Icon Out"=w360:picture)  [unwired: 7 out]
                      n92 = case shown="False" w356 {
                        tunnel: w360 -> [w376 w378]
                        tunnel: w359 -> [w375 w377]
                        tunnel: [w374 w378] -> w358
                        tunnel: [w373 w377] -> w357
                        frame False {
                          n93 = call "Rotate Flip Image.vi"("Rotate?"=TRUE, "rect"=w375, "Temp Icon In"=w376) -> ("rect out"=w373:T14, "Temp Icon Out"=w374:picture)  [unwired: 7 out]
                        }
                        frame True {
                        }
                      }
                      n94 = Bundle By Name(cluster=w369, "Image"=w358, "Rectangle"=w357) -> (w366:T13)
                      n95 = call "TemporaryGlyphView.vi"("Mouse Coords Pic"=w348, "Path & Icon"=w366) -> ("icon out"=w352:picture)  [unwired: 9 out]
                      n96 = call-dynamic "SET_ActiveGlyph.vi"("error in (no error)"=w367, "Active Glyph"=w366, "Glyph in"=w368) -> ("error out"=w349:errorcluster, "Glyph out"=w353:refnum<class "Glyph.lvclass">)  [unwired: 7 out]
                      n97 = Bundle By Name(cluster=w354, "Class.Glyph"=w353, "Support.Temp Icon"=w352) -> (w351:T2)
                    }
                  }
                }
                frame "Escape" {
                  n98 = call "IsAntsRectValid.vi"("AntsRect"=w388) -> ("Valid?"=w389:bool)  [unwired: 10 out]
                  n99 = Compound Arithmetic op=OR(w389, w387, w386, w385, w384) -> (w383:bool)
                  n100 = call "Escape.vi"("error in"=w391, "Data in"=w382) -> ("error out"=w379:errorcluster, "Data out"=w381:T2)  [unwired: 8 out]
                  n101 = call "Reset layer template selection.vi"("error in (no error)"=w379, "Data in"=w381) -> ("error out"=w390:errorcluster, "Data out"=w380:T2)  [unwired: 1 in, 7 out]
                }
                frame "Ctrl" {
                  n102 = Bundle By Name(cluster=w393, "Support.CTRL Pressed"=TRUE ("CTRL Pressed")) -> (w392:T2)
                }
              }
            }
            frame "Move Selection" {
              n103 = case shown="\"Delete\"" w406 {
                selector: w406 -> [_ w415 _ _]
                tunnel: w408 -> [w410 w413 w447 w456]
                tunnel: [w410 w412 w440 w463] -> w407
                tunnel: w405 -> [_ w417 w454 w455]
                tunnel: w404 -> [_ _ w452 _]
                tunnel: w403 -> [_ _ w451 _]
                tunnel: w402 -> [_ _ w450 _]
                tunnel: w401 -> [_ _ w449 _]
                tunnel: [_ _ w448 _] -> w400
                tunnel: w399 -> [w409 w419 w444 w457]
                tunnel: [w409 w416 w441 w461] -> w398
                tunnel: w397 -> [_ w411 w446 _]
                tunnel: w396 -> [_ w414 _ _]
                frame "ASCII", Default {
                }
                frame "Up".."Right" {
                  n104 = call "IsAntsRectValid.vi"("AntsRect"=w417) -> ("Valid?"=w418:bool)  [unwired: 10 out]
                  n105 = case shown="True" w418 {
                    tunnel: w419 -> [w421 w435]
                    tunnel: w417 -> [_ w424]
                    tunnel: [w421 w434] -> w416
                    tunnel: w415 -> [_ w428]
                    tunnel: w414 -> [_ w432]
                    tunnel: w413 -> [w420 w422]
                    tunnel: [w420 w427] -> w412
                    tunnel: w411 -> [_ w426]
                    frame False {
                    }
                    frame True {
                      n106 = case shown="\"Up\", Default" w428 {
                        tunnel: [T11 {"left"=0, "top"=-1, "right"=0, "bottom"=-1} ("y") T11 {"left"=0, "top"=1, "right"=0, "bottom"=1} ("y") T11 {"left"=-1, "top"=0, "right"=-1, "bottom"=0} ("y") T11 {"left"=1, "top"=0, "right"=1, "bottom"=0} ("y")] -> w433
                        frame "Up", Default {
                        }
                        frame "Down" {
                        }
                        frame "Left" {
                        }
                        frame "Right" {
                        }
                      }
                      n107 = Select(t=i16 3 ("left"), s=w432, f=i16 1 ("left")) -> (s? t:f=w429:i16)
                      n108 = Multiply(x=w433, y=w429) -> (x*y=w425:T11)
                      n109 = call "CheckBoundsAndIncrement.vi"("Increment"=w425, "Rectangle In"=w424) -> ("Rectangle Out"=w423:T11)  [unwired: 9 in]
                      n110 = Bundle By Name(cluster=w435, "Support.AntsRect"=w423) -> (w434:T2)
                      n111 = call "FireAntsEvent.vi"("error in (no error)"=w422, "Rectangle (default: deselect)"=w423, "Ants in"=w426) -> ("error out"=w427:errorcluster)  [unwired: 1 in, 7 out]
                    }
                  }
                }
                frame "Escape" {
                  n112 = call "IsAntsRectValid.vi"("AntsRect"=w454) -> ("Valid?"=w453:bool)  [unwired: 10 out]
                  n113 = Compound Arithmetic op=OR(w453, w452, w451, w450, w449) -> (w448:bool)
                  n114 = call "FireAntsEvent.vi"("error in (no error)"=w447, "Ants in"=w446) -> ("error out"=w445:errorcluster)  [unwired: 2 in, 7 out]
                  n115 = call "Reset layer template selection.vi"("error in (no error)"=w445, "Data in"=w444) -> ("error out"=w443:errorcluster, "Data out"=w442:T2)  [unwired: 1 in, 7 out]
                  n116 = call "Escape.vi"("error in"=w443, "Data in"=w442) -> ("error out"=w440:errorcluster, "Data out"=w441:T2)  [unwired: 8 out]
                }
                frame "Delete" {
                  n117 = call "IsAntsRectValid.vi"("AntsRect"=w455) -> ("Valid?"=w462:bool, "Max. Rect size?"=w458:bool)  [unwired: 9 out]
                  n118 = case shown="True" w458 {
                    tunnel: w462 -> [_ _]
                    tunnel: w457 -> [w473 w477]
                    tunnel: [w472 w484] -> w460
                    tunnel: [w471 w485] -> w459
                    tunnel: w456 -> [w464 w475]
                    tunnel: w455 -> [_ w483]
                    frame False {
                      w470 = TRUE ("Delete Selected Area?")
                      n119 = call "PrepareTemporaryView.vi"("Delete Selected Area?"=w470, "error in (no error)"=w464, "Valid Selection?"=w470, "Data in"=w473) -> ("error out"=w467:errorcluster, "Highlighted?"=w468:bool, "All Layers out"=w469:refnum<class "Layer.lvclass">[], "Data out"=w465:T2, "#Active Layer"=w466:i32)  [unwired: 1 in, 2 out]
                      n120 = call "Selection_SetNewData.vi"("#Active Layer"=w466, "error in"=w467, "Highlighted?"=w468, "All Layers In"=w469, "Data in"=w465) -> ("error out"=w472:errorcluster, "Data out"=w471:T2)  [unwired: 1 in, 3 out]
                    }
                    frame True {
                      n121 = Unbundle By Name(w477) -> ("Class.Icon"=w482:refnum<class "Icon.lvclass">)
                      n122 = call-dynamic "GET_All User Layers.vi"("error in (no error)"=w475, "Icon.lvclass in"=w482) -> ("error out"=w481:errorcluster, "User Layer"=w478:refnum<class "Layer.lvclass">[])  [unwired: 7 in, 1 out]
                      n123 = Array Size(array=w478) -> (size(s)=w479:i32)
                      n124 = for {
                        N: w479 -> [_]
                        tunnel: [w486] -> w480 mode=indexing
                        i -> [w486]
                      }
                      n125 = call "Set active Layer programmatically.vi"("error in"=w481, "Active Layer []"=w480, "Data in"=w477) -> ("error out"=w474:errorcluster, "Data out"=w476:T2)  [unwired: 7 in]
                      n126 = call "DeleteLayer.vi"("error in"=w474, "AntsRect"=w483, "Data in"=w476) -> ("error out"=w484:errorcluster, "Data out"=w485:T2)  [unwired: 5 out]
                    }
                  }
                  n127 = call "Escape.vi"("error in"=w460, "Data in"=w459) -> ("error out"=w463:errorcluster, "Data out"=w461:T2)  [unwired: 8 out]
                }
              }
            }
          }
        }
        frame True {
          n128 = Unbundle By Name(w505) -> ("Support.AntsRect"=w487:T11, "Support.Action"=w492:T7, "Support.Mouse Down?"=w501:bool, "Support.Mouse inside icon?"=w502:bool, "Ref.Tools"=w507:refnum<vi>)
          n129 = Equal?(x=lveventtype."Key Repeat", y=w498) -> (x = y?=w496:bool)
          n130 = Equal?(x=lveventtype."Key Repeat?", y=w498) -> (x = y?=w497:bool)
          n131 = Or(x=w496, y=w497) -> (x .or. y?=w495:bool)
          n132 = case shown="\"Tool\"" w492 {
            tunnel: w507 -> [_ w580 w672]
            tunnel: w506 -> [w512 w579 w675]
            tunnel: w505 -> [w514 w578 w680]
            tunnel: [w511 w577 w679] -> w504
            tunnel: [w510 w576 w674] -> w503
            tunnel: w502 -> [_ w575 _]
            tunnel: w501 -> [_ w574 _]
            tunnel: w494 -> [_ w573 w677]
            tunnel: w493 -> [_ w572 w673]
            tunnel: w491 -> [w513 w570 w678]
            tunnel: [w509 w569 w676] -> w489
            tunnel: w488 -> [w508 w568 _]
            tunnel: w487 -> [_ w567 _]
            frame "Default", Default {
              n133 = case shown="\"C\", \"c\"" w513 {
                tunnel: w514 -> [w523 w551 w558 w565]
                tunnel: w512 -> [w522 w550 w560 w566]
                tunnel: [w520 w551 w552 w561] -> w511
                tunnel: [w517 w550 w559 w562] -> w510
                tunnel: [w521 _ w556 w563] -> w509
                tunnel: w508 -> [w515 _ _ _]
                frame "V", "v" {
                  # "Paste"
                  n134 = call "IE Read from Clipboard.vi"("error in"=w522, "Data in"=w523) -> ("error out"=w518:errorcluster, "Key Focus"=w521:bool, "Data out"=w519:T2, "Empty Clipboard string?"=w516:bool)  [unwired: 6 in]
                  n135 = case shown="False" w516 {
                    tunnel: [w526 w533] -> w520
                    tunnel: w519 -> [w525 w534]
                    tunnel: w518 -> [w524 w536]
                    tunnel: [w524 w530] -> w517
                    tunnel: w515 -> [_ w529]
                    frame False {
                      w528 = u32 111  # Invalid tool value
                      w527 = FALSE ("Support.CTRL Pressed")
                      n136 = Bundle By Name(cluster=w525, "Support.Shift pressed?"=w527, "Support.CTRL Pressed"=w527, "Support.Tool (old value)"=w528) -> (w526:T2)
                    }
                    frame True {
                      n137 = call "Empty Picture"() -> ("empty picture"=w537:picture)
                      n138 = call "Import_Clipboard.vi"("error in (no error)"=w536, "Picture in"=w537) -> ("error out"=w532:errorcluster, "Valid?"=w535:bool, "Picture"=w531:picture)  [unwired: 1 in, 6 out]
                      n139 = case shown="True" w535 {
                        tunnel: w534 -> [w539 w547]
                        tunnel: [w539 w540] -> w533
                        tunnel: w532 -> [w538 w548]
                        tunnel: w531 -> [_ w549]
                        tunnel: [w538 w542] -> w530
                        tunnel: w529 -> [_ w543]
                        frame False {
                        }
                        frame True {
                          n140 = call "Create new layer_LayerName_Picture.vi"("error in"=w548, "Layer name"=w543, "Picture"=w549, "Data in"=w547) -> ("error out"=w546:errorcluster, "Data out"=w545:T2)  [unwired: 6 in]
                          n141 = call "ViewLayer.vi"("error in (no error)"=w546, "Data in"=w545) -> ("error out"=w544:errorcluster, "Data out"=w541:T2)  [unwired: 2 in, 6 out]
                          n142 = call "Set Undo Flag.vi"("error in"=w544, "Data in"=w541) -> ("error out"=w542:errorcluster, "Data out"=w540:T2)  [unwired: 8 in]
                        }
                      }
                    }
                  }
                }
                frame Default {
                }
                frame "C", "c" {
                  w555 = u32 111  # Invalid tool value
                  w554 = FALSE ("Support.CTRL Pressed")
                  n143 = call "IE Write to Clipboard.vi"("Is Cut?"=FALSE, "error in"=w560, "Data in"=w558) -> ("error out"=w559:errorcluster, "Key Focus"=w556:bool, "Data out"=w553:T2)  [unwired: 6 in]
                  n144 = Bundle By Name(cluster=w553, "Support.Shift pressed?"=w554, "Support.CTRL Pressed"=w554, "Support.Tool (old value)"=w555) -> (w552:T2)
                }
                frame "X", "x" {
                  n145 = call "IE Write to Clipboard.vi"("Is Cut?"=TRUE, "error in"=w566, "Data in"=w565) -> ("error out"=w562:errorcluster, "Key Focus"=w563:bool, "Data out"=w561:T2)  [unwired: 6 in]
                }
              }
            }
            frame "Tool" {
              n146 = Compound Arithmetic op=AND(invert w574, w575) -> (w571:bool)
              n147 = case shown="\"X\", \"x\"" w570 {
                tunnel: w580 -> [w593 _ _ _]
                tunnel: w579 -> [w592 w645 w663 w670]
                tunnel: w578 -> [w589 w649 w665 w671]
                tunnel: [w588 w647 w664 w666] -> w577
                tunnel: [w586 w648 w662 w668] -> w576
                tunnel: w571 -> [w585 _ _ _]
                tunnel: w573 -> [w584 _ _ _]
                tunnel: w572 -> [w583 _ _ _]
                tunnel: [_ w644 w660 w667] -> w569
                tunnel: w568 -> [_ w646 _ _]
                tunnel: w567 -> [w582 _ _ _]
                frame Default {
                  n148 = call "IsAntsRectValid.vi"("AntsRect"=w582) -> ("Valid?"=w581:bool)  [unwired: 10 out]
                  n149 = property class="RadioBtnsControl (strict)"(reference=w593, error in=w592) -> (reference out=w587:refnum<vi>, error out=w590:errorcluster, "Value"=w591:T12)
                  n150 = case shown="\"Select\"" w591 {
                    selector: w591 -> [w600 w619 _]
                    tunnel: w590 -> [w598 w622 w642]
                    tunnel: w589 -> [w602 w624 w643]
                    tunnel: [w601 w623 w641] -> w588
                    tunnel: w585 -> [w599 _ _]
                    tunnel: w587 -> [w597 w620 _]
                    tunnel: [w596 w621 w642] -> w586
                    tunnel: w584 -> [w595 w618 w640]
                    tunnel: w583 -> [w594 w617 w639]
                    tunnel: w581 -> [_ w625 _]
                    frame "Pencil", Default {
                      n151 = case shown="False" w599 {
                        tunnel: w602 -> [w607 w611]
                        tunnel: [w605 w616] -> w601
                        tunnel: w600 -> [_ w615]
                        tunnel: w598 -> [w606 w610]
                        tunnel: w597 -> [_ w614]
                        tunnel: [w606 w613] -> w596
                        tunnel: w595 -> [_ w609]
                        tunnel: w594 -> [_ w608]
                        frame False {
                          w604 = u32 111  # Invalid tool value
                          w603 = FALSE ("Support.CTRL Pressed")
                          n152 = Bundle By Name(cluster=w607, "Support.Shift pressed?"=w603, "Support.CTRL Pressed"=w603, "Support.Tool (old value)"=w604) -> (w605:T2)
                        }
                        frame True {
                          n153 = property class="RadioBtnsControl (strict)"(reference=w614, error in=w610, "Val(Sgnl)"=T12."Dropper" ("Value (Signaling)")) -> (error out=w613:errorcluster)  [unwired: 1 out]
                          n154 = Bundle By Name(cluster=w611, "Support.Tool (old value)"=w615, "Support.Shift pressed?"=w609, "Support.CTRL Pressed"=w608) -> (w616:T2)
                        }
                      }
                    }
                    frame "Select" {
                      n155 = case shown="True" w625 {
                        tunnel: w624 -> [w630 w638]
                        tunnel: [w629 w636] -> w623
                        tunnel: w622 -> [w633 w637]
                        tunnel: [w632 w637] -> w621
                        tunnel: w620 -> [w631 _]
                        tunnel: w619 -> [w628 _]
                        tunnel: w618 -> [w627 _]
                        tunnel: w617 -> [w626 _]
                        frame False {
                          n156 = Bundle By Name(cluster=w630, "Support.Tool (old value)"=w628, "Support.Shift pressed?"=w627, "Support.CTRL Pressed"=w626) -> (w629:T2)
                          n157 = property class="RadioBtnsControl (strict)"(reference=w631, error in=w633, "Val(Sgnl)"=T12."Dropper" ("Value (Signaling)")) -> (error out=w632:errorcluster)  [unwired: 1 out]
                        }
                        frame True {
                          w635 = u32 111  # Invalid tool value
                          n158 = Bundle By Name(cluster=w638, "Support.Tool (old value)"=w635) -> (w636:T2)
                        }
                      }
                    }
                    frame "Dropper" {
                      n159 = Bundle By Name(cluster=w643, "Support.Shift pressed?"=w640, "Support.CTRL Pressed"=w639) -> (w641:T2)
                    }
                  }
                }
                frame "V", "v" {
                  n160 = call "IE Read from Clipboard.vi"("error in"=w645, "Data in"=w649) -> ("error out"=w651:errorcluster, "Key Focus"=w644:bool, "Data out"=w652:T2, "Empty Clipboard string?"=w650:bool)  [unwired: 6 in]
                  n161 = case shown="False" w650 {
                    tunnel: [w655 w658] -> w647
                    tunnel: w652 -> [w654 w658]
                    tunnel: w651 -> [w653 w659]
                    tunnel: [w653 w659] -> w648
                    tunnel: w646 -> [_ _]
                    frame False {
                      w657 = u32 111  # Invalid tool value
                      w656 = FALSE ("Support.CTRL Pressed")
                      n162 = Bundle By Name(cluster=w654, "Support.Shift pressed?"=w656, "Support.CTRL Pressed"=w656, "Support.Tool (old value)"=w657) -> (w655:T2)
                    }
                    frame True {
                    }
                  }
                }
                frame "C", "c" {
                  n163 = call "IE Write to Clipboard.vi"("Is Cut?"=FALSE, "error in"=w663, "Data in"=w665) -> ("error out"=w662:errorcluster, "Key Focus"=w660:bool, "Data out"=w664:T2)  [unwired: 6 in]
                }
                frame "X", "x" {
                  n164 = call "IE Write to Clipboard.vi"("Is Cut?"=TRUE, "error in"=w670, "Data in"=w671) -> ("error out"=w668:errorcluster, "Key Focus"=w667:bool, "Data out"=w666:T2)  [unwired: 6 in]
                }
              }
            }
            frame "Move Selection" {
              n165 = case shown="\"Z\", \"z\"" w678 {
                tunnel: w675 -> [w681 w688 w700]
                tunnel: w680 -> [w682 w687 w701]
                tunnel: [w682 w686 w698] -> w679
                tunnel: w677 -> [_ w685 _]
                tunnel: [_ w684 _] -> w676
                tunnel: [w681 w683 w699] -> w674
                tunnel: w673 -> [_ _ _]
                tunnel: w672 -> [_ _ _]
                frame Default {
                }
                frame "Z", "z" {
                  n166 = case shown="False" w685 {
                    tunnel: w688 -> [w692 w695]
                    tunnel: w687 -> [w694 w697]
                    tunnel: [w693 w697] -> w686
                    tunnel: [TRUE TRUE] -> w684
                    tunnel: [w691 w695] -> w683
                    frame False {
                      n167 = call "Escape.vi"("Reset cursor (T)"=FALSE, "error in"=w692, "Data in"=w694) -> ("error out"=w691:errorcluster, "Data out"=w693:T2)  [unwired: 7 out]
                    }
                    frame True {
                    }
                  }
                }
                frame "V", "v" {
                  n168 = call "Finalize Movement.vi"("error in (no error)"=w700, "Data in"=w701) -> ("error out"=w699:errorcluster, "Data out"=w698:T2)  [unwired: 2 in, 6 out]
                }
              }
            }
          }
          n169 = Or(x=w489, y=w495) -> (x .or. y?=w490:bool)
        }
      }
    }
    frame Error {
    }
  }
  "error out" <- w9
  "Discard?" <- w5
  "Data out" <- w3
